vi "MultiParamGrid.vi"() -> ()   [LabVIEW 2014]
uses:
  <userlib>/Nanonis Prog Interface V5/Nanonis Prog Interface.lvlib
panel:
  out "set value":dbl format="%#_6p"
  out "next value":dbl=2e-10 format="%#_6p"
  out "waited:":i32=20000 format="%.0p"
  out "Grid Running?":bool=TRUE
  out "Values":i32(listbox)
  in  "External VI path":path=path "D:/Scripts/VIs/Topo & GridSpectr_DriftCorrection_zSpec_v19.vi"
  in  "engage":bool=TRUE
  in  "Control Name":string="STS z offset"
  # "Zero is \"0\""
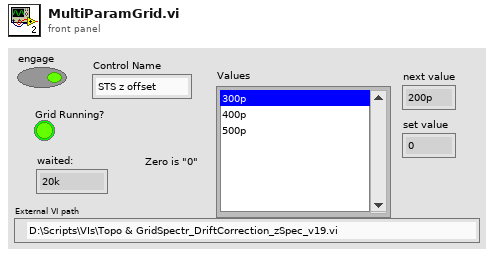
[diagram p1: front panel]
types:
  T1 = enum16{"Header", "TOPO", "STS", "GRID", "GRIDCloud"}
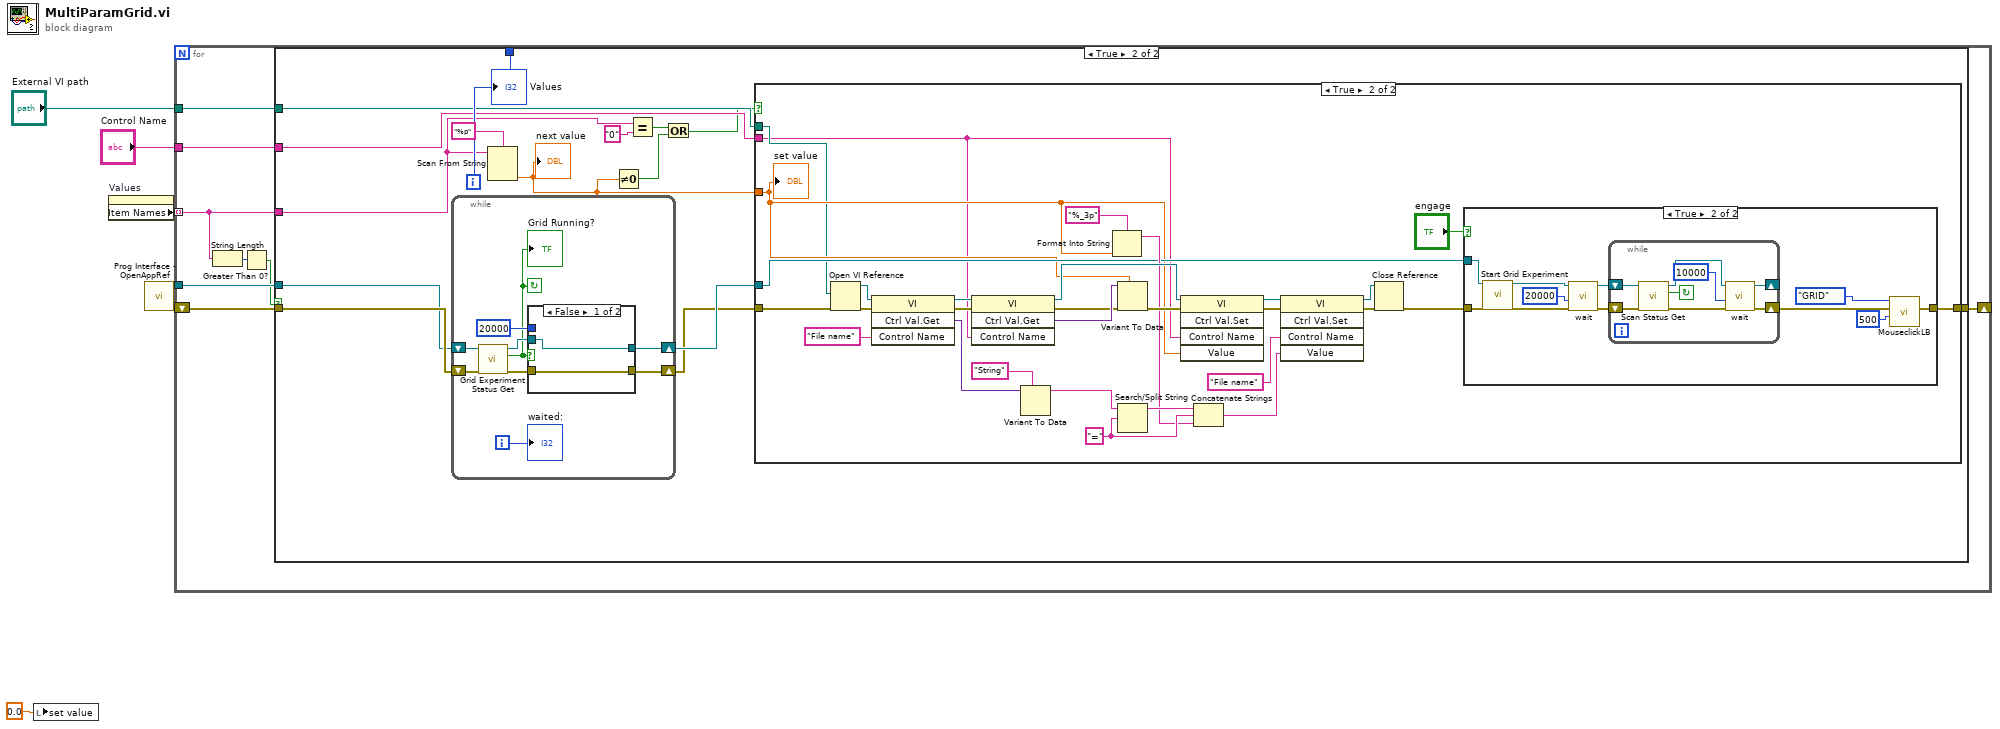
[diagram p0: block diagram]
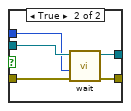
[diagram p5: hidden frame]
diagram:
  n1 = local write "set value"(0.0 ("set value")) -> ()
  n2 = property on="Values" class="LstBox (strict)"() -> ("Item Names"=w4:string[])  [unwired: 2 in, 2 out]
  n3 = call <userlib>:"Prog Interface - OpenAppRef.vi"() -> ("Error out"=w6:errorcluster, "Application reference"=w5:refnum<vi>)  [unwired: 6 in]
  n4 = for {
    tunnel: w5 -> [w14]
    tunnel: w4 -> [w9] mode=indexing
    tunnel: "External VI path" -> [w12]
    tunnel: "Control Name" -> [w11]
    shift-right: [w10] -> _
    shift-left: w6 -> [w15]
    i -> [w13]
    n5 = String Length(string=w9) -> (length=w8:i32)
    n6 = Greater Than 0?(x=w8) -> (x > 0?=w7:bool)
    n7 = case shown="True" w7 {
      tunnel: w15 -> [w16 w31]
      tunnel: w14 -> [_ w30]
      tunnel: w13 -> [_ w26]
      tunnel: w9 -> [_ w23]
      tunnel: w12 -> [_ w20]
      tunnel: w11 -> [_ w19]
      tunnel: [w16 w18] -> w10
      frame False {
      }
      frame True {
        n8 = while {
          shift-right: [w88] -> w29
          shift-left: w30 -> [w90]
          shift-right: [w87] -> w28
          shift-left: w31 -> [w91]
          i -> [w84]
          stop <- w83 continue-if-true
          n9 = call <userlib>:"Grid Experiment Status Get.vi"("error in (no error)"=w91, "Application ref in"=w90) -> ("error out"=w86:errorcluster, "Running?"=w83:bool, "Application ref out"=w89:refnum<vi>)  [unwired: 7 in]
          "Grid Running?" <- w83
          n10 = case shown="False" w83 {
            tunnel: w89 -> [w93 w98]
            tunnel: [w93 w97] -> w88
            tunnel: [w92 w96] -> w87
            tunnel: w86 -> [w92 w95]
            tunnel: u32 20000 ("milliseconds to wait") -> [_ w94]
            frame False {
            }
            frame True {
              n11 = call "wait.vi"("error in"=w95, "milliseconds to wait"=w94, "application reference in"=w98) -> ("error out"=w96:errorcluster, "application reference out"=w97:refnum<vi>)  [unwired: 7 in]
            }
          }
          "waited:" <- w84
        }
        n12 = Scan From String(format string="%p", input string=w23) -> (output 1=w21:dbl)  [unwired: 3 in, 3 out]
        "next value" <- w21
        n13 = Not Equal To 0?(x=w21) -> (x != 0?=w22:bool)
        n14 = Equal?(x=w23, y="0") -> (x = y?=w24:bool)
        n15 = Or(x=w24, y=w22) -> (x .or. y?=w17:bool)
        n16 = case shown="True" w17 {
          tunnel: w29 -> [_ w38]
          tunnel: w28 -> [w32 w37]
          tunnel: w21 -> [_ w36]
          tunnel: w20 -> [_ w35]
          tunnel: w19 -> [_ w34]
          tunnel: [w32 w33] -> w18
          frame False {
          }
          frame True {
            w43 = "=" ("search string")
            n17 = Open VI Reference(vi path=w35, error in (no error)=w37) -> (vi reference=w57:refnum<vi>, error out=w56:errorcluster)  [unwired: 4 in]
            n18 = invoke class="VI" method="Ctrl Val.Get"(reference=w57, error in=w56, "Control Name"="File name") -> (reference out=w55:refnum<vi>, error out=w54:errorcluster, "Get Control Value Variant"=w47:variant)  [unwired: 1 in, 1 out]
            n19 = invoke class="VI" method="Ctrl Val.Get"(reference=w55, error in=w54, "Control Name"=w34) -> (reference out=w62:refnum<vi>, error out=w60:errorcluster, "Get Control Value Variant"=w61:variant)  [unwired: 1 in, 1 out]
            n20 = Variant To Data(type="String" ("Control Name"), Variant=w47) -> (data=w45:string)  [unwired: 1 in, 1 out]
            n21 = Format Into String(format string="%_3p", w36) -> (resulting string=w41:string)  [unwired: 2 in, 1 out]
            n22 = Variant To Data(error in=w60, type=w36, Variant=w61) -> (error out=w59:errorcluster)  [unwired: 1 out]
            n23 = Search/Split String(string=w45, search string/char (-)=w43) -> (substring before match=w42:string)  [unwired: 1 in, 2 out]
            n24 = invoke class="VI" method="Ctrl Val.Set"(reference=w62, error in=w59, "Control Name"=w34, "Value"=w36) -> (reference out=w53:refnum<vi>, error out=w52:errorcluster)  [unwired: 1 in, 3 out]
            n25 = Concatenate Strings(w42, w43, w41) -> (w40:string)
            n26 = invoke class="VI" method="Ctrl Val.Set"(reference=w53, error in=w52, "Control Name"="File name", "Value"=w40) -> (reference out=w51:refnum<vi>, error out=w50:errorcluster)  [unwired: 1 in, 3 out]
            n27 = Close Reference(reference=w51, error in (no error)=w50) -> (error out=w58:errorcluster)
            n28 = case shown="True" "engage" {
              tunnel: w58 -> [w63 w74]
              tunnel: w38 -> [_ w73]
              tunnel: [w63 w66] -> w33
              frame False {
              }
              frame True {
                n29 = call <userlib>:"Start Grid Experiment.vi"("Application ref in"=w73, "error in (no error)"=w74) -> ("Application ref out"=w72:refnum<vi>, "error out"=w71:errorcluster)  [unwired: 16 in]
                n30 = call "wait.vi"("error in"=w71, "milliseconds to wait"=u32 20000, "application reference in"=w72) -> ("error out"=w70:errorcluster, "application reference out"=w69:refnum<vi>)  [unwired: 7 in]
                n31 = while {
                  shift-right: [w75] -> w67
                  shift-left: w70 -> [w81]
                  shift-right: [w76] -> _
                  shift-left: w69 -> [w82]
                  stop <- w80 continue-if-true
                  n32 = call <userlib>:"Scan Status Get.vi"("error in (no error)"=w81, "Application ref in"=w82) -> ("error out"=w79:errorcluster, "Scanning?"=w80:bool, "Application ref out"=w78:refnum<vi>)  [unwired: 6 in]
                  n33 = call "wait.vi"("error in"=w79, "milliseconds to wait"=u32 10000, "application reference in"=w78) -> ("error out"=w75:errorcluster, "application reference out"=w76:refnum<vi>)  [unwired: 7 in]
                }
                n34 = call "MouseclickLB.vi"("nMilliseconds"=500, "error in (no error)"=w67, "Click"=T1."GRID") -> ("error out"=w66:errorcluster)  [unwired: 8 in]
              }
            }
            "set value" <- w36
          }
        }
        "Values" <- w26
      }
    }
  }
